vi "Open CANCoders.vi"(8 "error in":errorcluster) -> (0 "error out":errorcluster, 3 "output cluster":T2)   [LabVIEW 2020]
uses:
  <vilib>/Rock Robotics/WPI/ThirdParty/Phoenix-LabVIEW/CANCoder/Controls/CTRE_Phoenix_CANcoder_DeviceRef.ctl
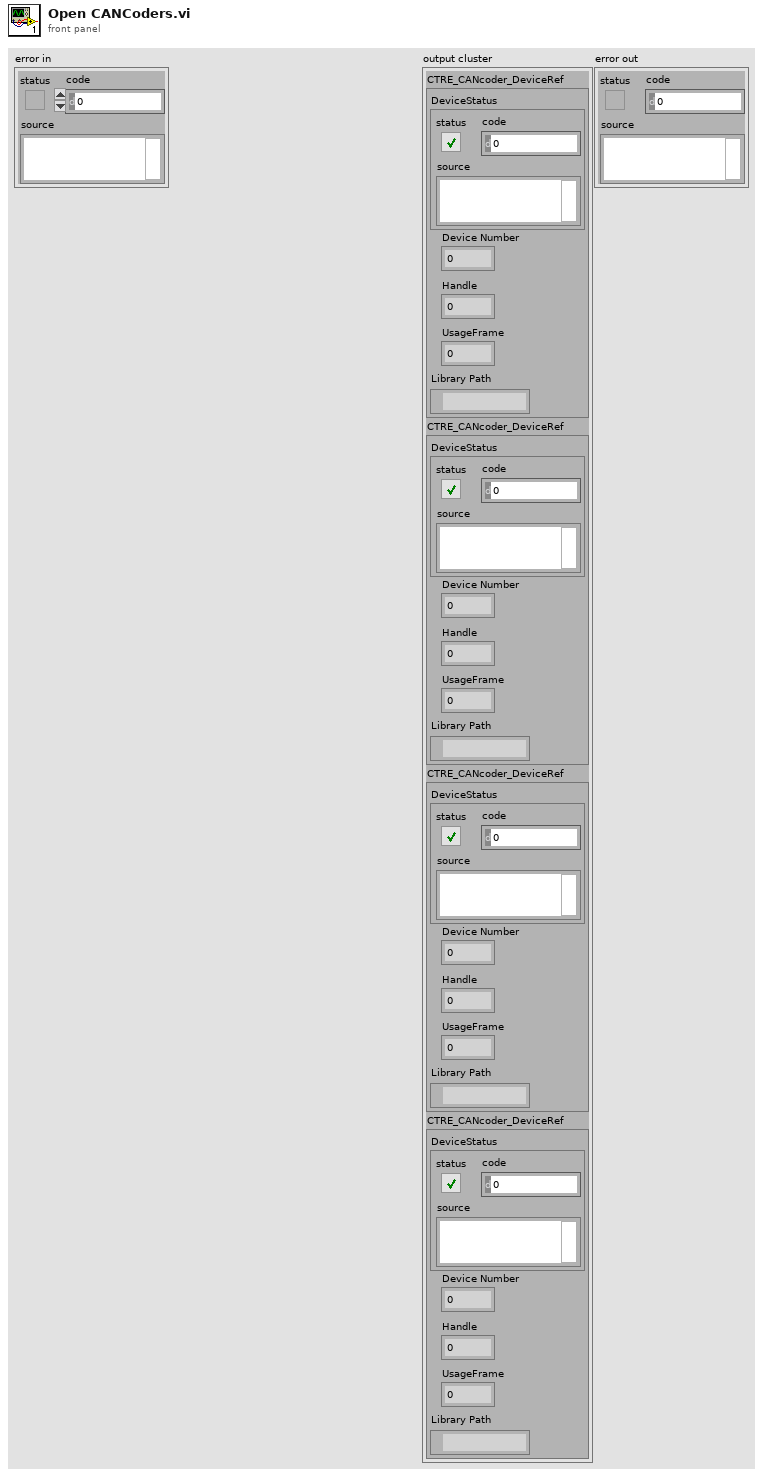
[diagram p1: front panel]
types:
  T1 = typedef "CTRE_Phoenix_CANcoder_DeviceRef.ctl" = cluster{"DeviceStatus":errorcluster, "Device Number":u8, "Handle":u64, "UsageFrame":u32, "Library Path":path}
  T2 = cluster{"CTRE_CANcoder_DeviceRef":T1, "CTRE_CANcoder_DeviceRef":T1, "CTRE_CANcoder_DeviceRef":T1, "CTRE_CANcoder_DeviceRef":T1}
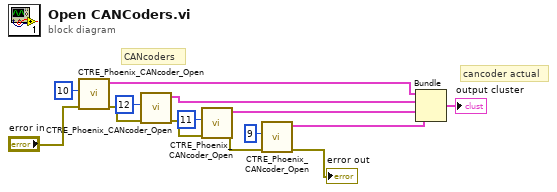
[diagram p0: block diagram]
diagram:
  # "CANcoders"
  # "cancoder actual"
  n1 = call <vilib>:"CTRE_Phoenix_CANcoder_Open.vi"("error in"="error in", "Device Number"=u8 10) -> ("error out"=w10:errorcluster, "CTRE_CANcoder_DeviceRef"=w8:T1)  [unwired: 8 in]
  n2 = call <vilib>:"CTRE_Phoenix_CANcoder_Open.vi"("error in"=w10, "Device Number"=u8 12) -> ("error out"=w9:errorcluster, "CTRE_CANcoder_DeviceRef"=w7:T1)  [unwired: 8 in]
  n3 = call <vilib>:"CTRE_Phoenix_CANcoder_Open.vi"("error in"=w9, "Device Number"=u8 11) -> ("error out"=w2:errorcluster, "CTRE_CANcoder_DeviceRef"=w6:T1)  [unwired: 8 in]
  n4 = call <vilib>:"CTRE_Phoenix_CANcoder_Open.vi"("error in"=w2, "Device Number"=u8 9) -> ("error out"=→"error out":errorcluster, "CTRE_CANcoder_DeviceRef"=w5:T1)  [unwired: 8 in]
  n5 = Bundle("CTRE_CANcoder_DeviceRef"=w8, "CTRE_CANcoder_DeviceRef"=w7, "CTRE_CANcoder_DeviceRef"=w6, "CTRE_CANcoder_DeviceRef"=w5) -> (→"output cluster":T2)  [unwired: 1 in]
